vi "publish node.vi"(8 "Error In":errorcluster, 9 "parent opcua path":string, 10 "OPC UA server refnum in":refnum<k21>, 11 "DOM node":refnum<k20>) -> (0 "Error Out":errorcluster, 2 "OPC UA server refnum out":refnum<k21>, 3 "DOM node (dup)":refnum<k20>)   [LabVIEW 2013]
uses:
  <resource>/objmgr/DOMUserDefRef.rc
  <vilib>/xml/NI_XML.lvlib
  <vilib>/xml/Close Reference(Node).vi
  <vilib>/OPCUA/NI OPC UA Server.lvlib
  <vilib>/xml/Close Reference(NNMap).vi
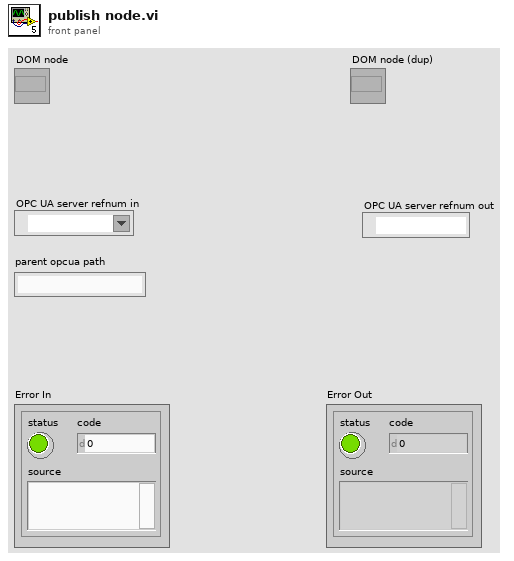
[diagram p1: front panel]
types:
  T1 = cluster{"name":string, "data type":u16, "access level":u16, "description":string}
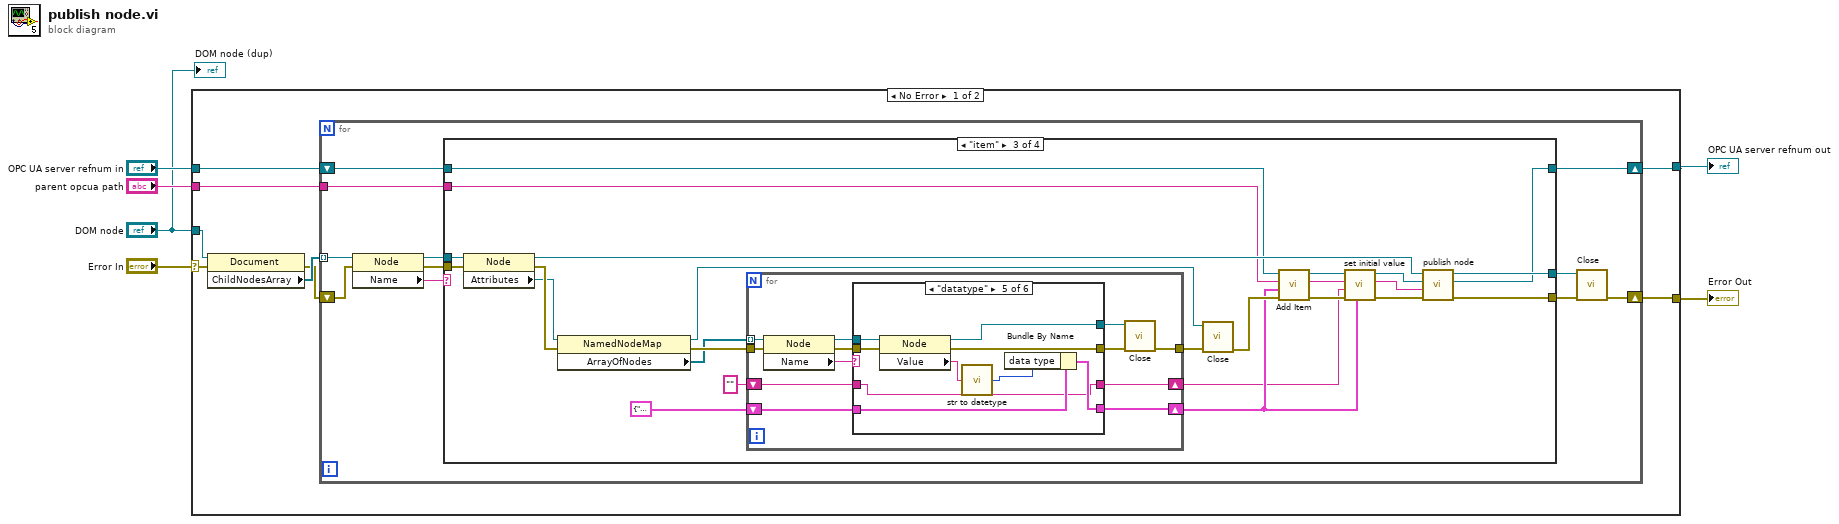
[diagram p0: block diagram]
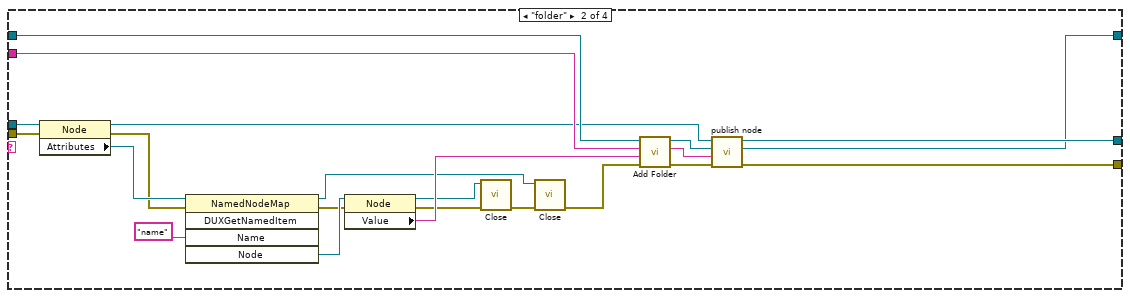
[diagram p3: hidden frame]
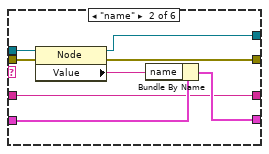
[diagram p5: hidden frame]
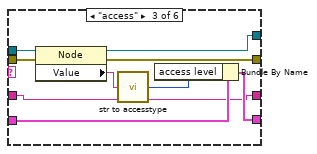
[diagram p6: hidden frame]
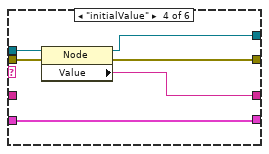
[diagram p7: hidden frame]
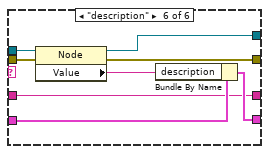
[diagram p8: hidden frame]
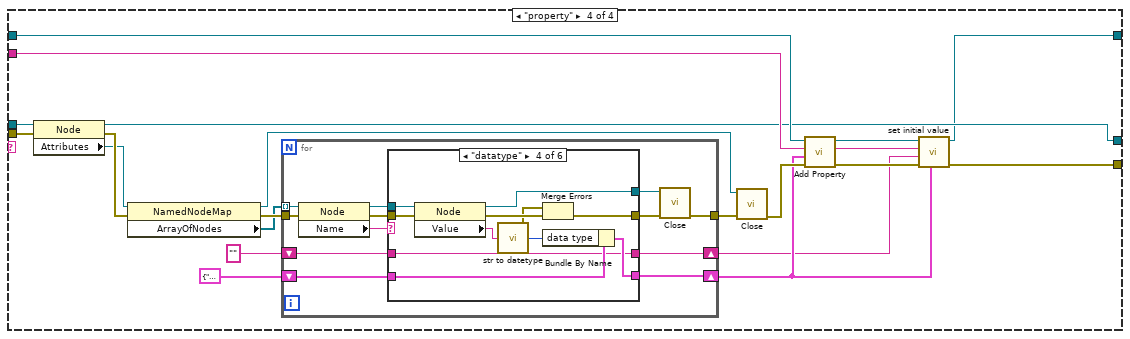
[diagram p9: hidden frame]
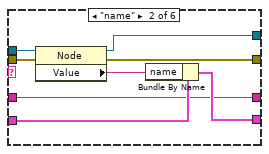
[diagram p11: hidden frame]
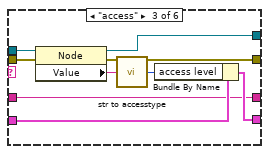
[diagram p12: hidden frame]
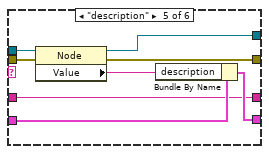
[diagram p13: hidden frame]
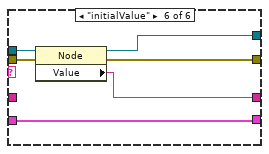
[diagram p14: hidden frame]
diagram:
  n1 = case shown="No Error" "Error In" {
    selector: "Error In" -> [w8 w212]
    tunnel: [w12 w212] -> w6
    tunnel: "DOM node" -> [w14 _]
    tunnel: "parent opcua path" -> [w11 _]
    tunnel: "OPC UA server refnum in" -> [w10 w211]
    tunnel: [w9 w211] -> w2
    frame No Error {
      n2 = property class="Document"(reference=w14, error in=w8) -> (error out=w7:errorcluster, "ChildNodesArray"=w13:refnum<k20>[])  [unwired: 1 out]
      n3 = for {
        tunnel: w13 -> [w25] mode=indexing
        shift-right: [w21] -> w12
        shift-left: w7 -> [w22]
        tunnel: w11 -> [w20]
        shift-right: [w18] -> w9
        shift-left: w10 -> [w19]
        n4 = property class="Node"(reference=w25, error in=w22) -> (reference out=w23:refnum<k20>, error out=w17:errorcluster, "Name"=w24:string)
        n5 = case shown="\"item\"" w24 {
          tunnel: w23 -> [w27 w50 w75 w143]
          tunnel: w20 -> [_ w46 w71 w151]
          tunnel: w19 -> [w26 w45 w72 w152]
          tunnel: [w26 w39 w70 w137] -> w18
          tunnel: w17 -> [w28 w36 w68 w142]
          tunnel: [w27 w42 w74 w141] -> w16
          tunnel: [w28 w41 w69 w136] -> w15
          frame Default {
          }
          frame "folder" {
            n6 = property class="Node"(reference=w50, error in=w36) -> (reference out=w43:refnum<k20>, error out=w35:errorcluster, "Attributes"=w49:refnum<k20>)
            n7 = invoke class="NamedNodeMap" method="DUXGetNamedItem"(reference=w49, error in=w35, "Name"="name") -> (reference out=w30:refnum<k20>, error out=w34:errorcluster, "Node"=w47:refnum<k20>)  [unwired: 2 in, 2 out]
            n8 = property class="Node"(reference=w47, error in=w34) -> (reference out=w29:refnum<k20>, error out=w33:errorcluster, "Value"=w44:string)
            n9 = call-poly <vilib>:"Close.vi"("error in (no error)"=w33, "node"=w29) -> ("error out"=w32:errorcluster)  [unwired: 7 out]
            n10 = call-poly <vilib>:"Close.vi"("error in (no error)"=w32, "named node map"=w30) -> ("error out"=w31:errorcluster)  [unwired: 7 out]
            n11 = call <vilib>:"Add Folder.vi"("error in (no error)"=w31, "folder name"=w44, "parent folder path"=w46, "OPC UA server refnum in"=w45) -> ("error out"=w37:errorcluster, "folder path"=w38:string, "OPC UA server refnum out"=w40:refnum<k21>)  [unwired: 4 in]
            n12 = call "publish node.vi"("Error In"=w37, "parent opcua path"=w38, "OPC UA server refnum in"=w40, "DOM node"=w43) -> ("Error Out"=w41:errorcluster, "OPC UA server refnum out"=w39:refnum<k21>, "DOM node (dup)"=w42:refnum<k20>)  [unwired: 5 in]
          }
          frame "item" {
            n13 = property class="Node"(reference=w75, error in=w68) -> (reference out=w73:refnum<k20>, error out=w67:errorcluster, "Attributes"=w66:refnum<k20>)
            n14 = property class="NamedNodeMap"(reference=w66, error in=w67) -> (reference out=w61:refnum<k20>, error out=w65:errorcluster, "ArrayOfNodes"=w64:refnum<k20>[])
            n15 = for {
              tunnel: [w84] -> w62
              tunnel: w65 -> [w87]
              tunnel: w64 -> [w86] mode=indexing
              shift-right: [w78] -> w53
              shift-left: T1 {"name"="", "data type"=1, "access level"=1, "description"=""} ("item") -> [w79]
              shift-right: [w77] -> w51
              shift-left: "" ("Value") -> [w76]
              n16 = property class="Node"(reference=w86, error in=w87) -> (reference out=w80:refnum<k20>, error out=w83:errorcluster, "Name"=w85:string)
              n17 = case shown="\"datatype\"" w85 {
                tunnel: [w90 w98 w107 w110 w122 w130] -> w82
                tunnel: w83 -> [w90 w99 w108 w112 w123 w131]
                tunnel: [w91 w97 w106 w111 w121 w129] -> w81
                tunnel: w80 -> [w91 w96 w105 w113 w120 w128]
                tunnel: w79 -> [w88 w94 w104 w114 w119 w127]
                tunnel: [w88 w93 w103 w114 w118 w126] -> w78
                tunnel: [w89 w92 w100 w109 w115 w124] -> w77
                tunnel: w76 -> [w89 w92 w100 _ w115 w124]
                frame Default {
                }
                frame "name" {
                  n18 = property class="Node"(reference=w96, error in=w99) -> (reference out=w97:refnum<k20>, error out=w98:errorcluster, "Value"=w95:string)
                  n19 = Bundle By Name(cluster=w94, "name"=w95) -> (w93:T1)
                }
                frame "access" {
                  n20 = property class="Node"(reference=w105, error in=w108) -> (reference out=w106:refnum<k20>, error out=w107:errorcluster, "Value"=w102:string)
                  n21 = call "str to accesstype.vi"("String"=w102) -> ("access level"=w101:u16)  [unwired: 6 in]
                  n22 = Bundle By Name(cluster=w104, "access level"=w101) -> (w103:T1)
                }
                frame "initialValue" {
                  n23 = property class="Node"(reference=w113, error in=w112) -> (reference out=w111:refnum<k20>, error out=w110:errorcluster, "Value"=w109:string)
                }
                frame "datatype" {
                  n24 = property class="Node"(reference=w120, error in=w123) -> (reference out=w121:refnum<k20>, error out=w122:errorcluster, "Value"=w116:string)
                  n25 = call "str to datetype.vi"("String"=w116) -> ("data type"=w117:u16)  [unwired: 5 in, 1 out]
                  n26 = Bundle By Name(cluster=w119, "data type"=w117) -> (w118:T1)
                }
                frame "description" {
                  n27 = property class="Node"(reference=w128, error in=w131) -> (reference out=w129:refnum<k20>, error out=w130:errorcluster, "Value"=w125:string)
                  n28 = Bundle By Name(cluster=w127, "description"=w125) -> (w126:T1)
                }
              }
              n29 = call-poly <vilib>:"Close.vi"("error in (no error)"=w82, "node"=w81) -> ("error out"=w84:errorcluster)  [unwired: 7 out]
            }
            n30 = call-poly <vilib>:"Close.vi"("error in (no error)"=w62, "named node map"=w61) -> ("error out"=w60:errorcluster)  [unwired: 7 out]
            n31 = call <vilib>:"Add Item.vi"("error in (no error)"=w60, "item"=w53, "parent folder path"=w71, "OPC UA server refnum in"=w72) -> ("error out"=w57:errorcluster, "item path"=w58:string, "OPC UA server refnum out"=w59:refnum<k21>)  [unwired: 4 in]
            n32 = call "set initial value.vi"("item"=w53, "Error In"=w57, "value string"=w51, "node path"=w58, "OPC UA server refnum in"=w59) -> ("Error Out"=w56:errorcluster, "node path (dup)"=w54:string, "OPC UA server refnum out"=w55:refnum<k21>)  [unwired: 4 in]
            n33 = call "publish node.vi"("Error In"=w56, "parent opcua path"=w54, "OPC UA server refnum in"=w55, "DOM node"=w73) -> ("Error Out"=w69:errorcluster, "OPC UA server refnum out"=w70:refnum<k21>, "DOM node (dup)"=w74:refnum<k20>)  [unwired: 5 in]
          }
          frame "property" {
            n34 = property class="Node"(reference=w143, error in=w142) -> (reference out=w141:refnum<k20>, error out=w150:errorcluster, "Attributes"=w149:refnum<k20>)
            n35 = property class="NamedNodeMap"(reference=w149, error in=w150) -> (reference out=w144:refnum<k20>, error out=w148:errorcluster, "ArrayOfNodes"=w147:refnum<k20>[])
            n36 = for {
              tunnel: [w161] -> w145
              tunnel: w148 -> [w164]
              tunnel: w147 -> [w163] mode=indexing
              shift-right: [w155] -> w134
              shift-left: T1 {"name"="", "data type"=1, "access level"=1, "description"=""} ("item") -> [w156]
              shift-right: [w153] -> w132
              shift-left: "" ("Node Value") -> [w154]
              n37 = property class="Node"(reference=w163, error in=w164) -> (reference out=w157:refnum<k20>, error out=w160:errorcluster, "Name"=w162:string)
              n38 = case shown="\"datatype\"" w162 {
                tunnel: [w166 w175 w184 w187 w203 w209] -> w159
                tunnel: w160 -> [w166 w176 w185 w196 w204 w210]
                tunnel: [w167 w174 w183 w194 w202 w208] -> w158
                tunnel: w157 -> [w167 w173 w182 w193 w201 w207]
                tunnel: w156 -> [w168 w171 w181 w192 w200 w206]
                tunnel: [w168 w170 w180 w191 w199 w206] -> w155
                tunnel: w154 -> [w165 w169 w177 w188 w197 _]
                tunnel: [w165 w169 w177 w188 w197 w205] -> w153
                frame Default {
                }
                frame "name" {
                  n39 = property class="Node"(reference=w173, error in=w176) -> (reference out=w174:refnum<k20>, error out=w175:errorcluster, "Value"=w172:string)
                  n40 = Bundle By Name(cluster=w171, "name"=w172) -> (w170:T1)
                }
                frame "access" {
                  n41 = property class="Node"(reference=w182, error in=w185) -> (reference out=w183:refnum<k20>, error out=w184:errorcluster, "Value"=w179:string)
                  n42 = call "str to accesstype.vi"("String"=w179) -> ("access level"=w178:u16)  [unwired: 6 in]
                  n43 = Bundle By Name(cluster=w181, "access level"=w178) -> (w180:T1)
                }
                frame "datatype" {
                  n44 = property class="Node"(reference=w193, error in=w196) -> (reference out=w194:refnum<k20>, error out=w195:errorcluster, "Value"=w189:string)
                  n45 = call "str to datetype.vi"("String"=w189) -> ("error out"=w186:errorcluster, "data type"=w190:u16)  [unwired: 5 in]
                  n46 = Merge Errors(w186, w195) -> (w187:errorcluster)
                  n47 = Bundle By Name(cluster=w192, "data type"=w190) -> (w191:T1)
                }
                frame "description" {
                  n48 = property class="Node"(reference=w201, error in=w204) -> (reference out=w202:refnum<k20>, error out=w203:errorcluster, "Value"=w198:string)
                  n49 = Bundle By Name(cluster=w200, "description"=w198) -> (w199:T1)
                }
                frame "initialValue" {
                  n50 = property class="Node"(reference=w207, error in=w210) -> (reference out=w208:refnum<k20>, error out=w209:errorcluster, "Value"=w205:string)
                }
              }
              n51 = call-poly <vilib>:"Close.vi"("error in (no error)"=w159, "node"=w158) -> ("error out"=w161:errorcluster)  [unwired: 7 out]
            }
            n52 = call-poly <vilib>:"Close.vi"("error in (no error)"=w145, "named node map"=w144) -> ("error out"=w140:errorcluster)  [unwired: 7 out]
            n53 = call <vilib>:"Add Property.vi"("error in (no error)"=w140, "property"=w134, "item path"=w151, "OPC UA server refnum in"=w152) -> ("error out"=w138:errorcluster, "property path"=w135:string, "OPC UA server refnum out"=w139:refnum<k21>)  [unwired: 4 in]
            n54 = call "set initial value.vi"("item"=w134, "Error In"=w138, "value string"=w132, "node path"=w135, "OPC UA server refnum in"=w139) -> ("Error Out"=w136:errorcluster, "OPC UA server refnum out"=w137:refnum<k21>)  [unwired: 4 in, 1 out]
          }
        }
        n55 = call-poly <vilib>:"Close.vi"("error in (no error)"=w15, "node"=w16) -> ("error out"=w21:errorcluster)  [unwired: 7 out]
      }
    }
    frame Error {
    }
  }
  "Error Out" <- w6
  "OPC UA server refnum out" <- w2
  "DOM node (dup)" <- "DOM node"
